vi "save.comics.vi"(8 "error in":errorcluster, 11 "data":T1) -> (0 "error out":errorcluster)   [LabVIEW 2024]
uses:
  TypeDefs/comics.reply--cluster.ctl
  TypeDefs/comic--cluster.ctl
  <vilib>/addons/_JKI.lib/Serialization/JSON/JKI JSON Serialization.lvlib
panel:
  out "all lower case string":string
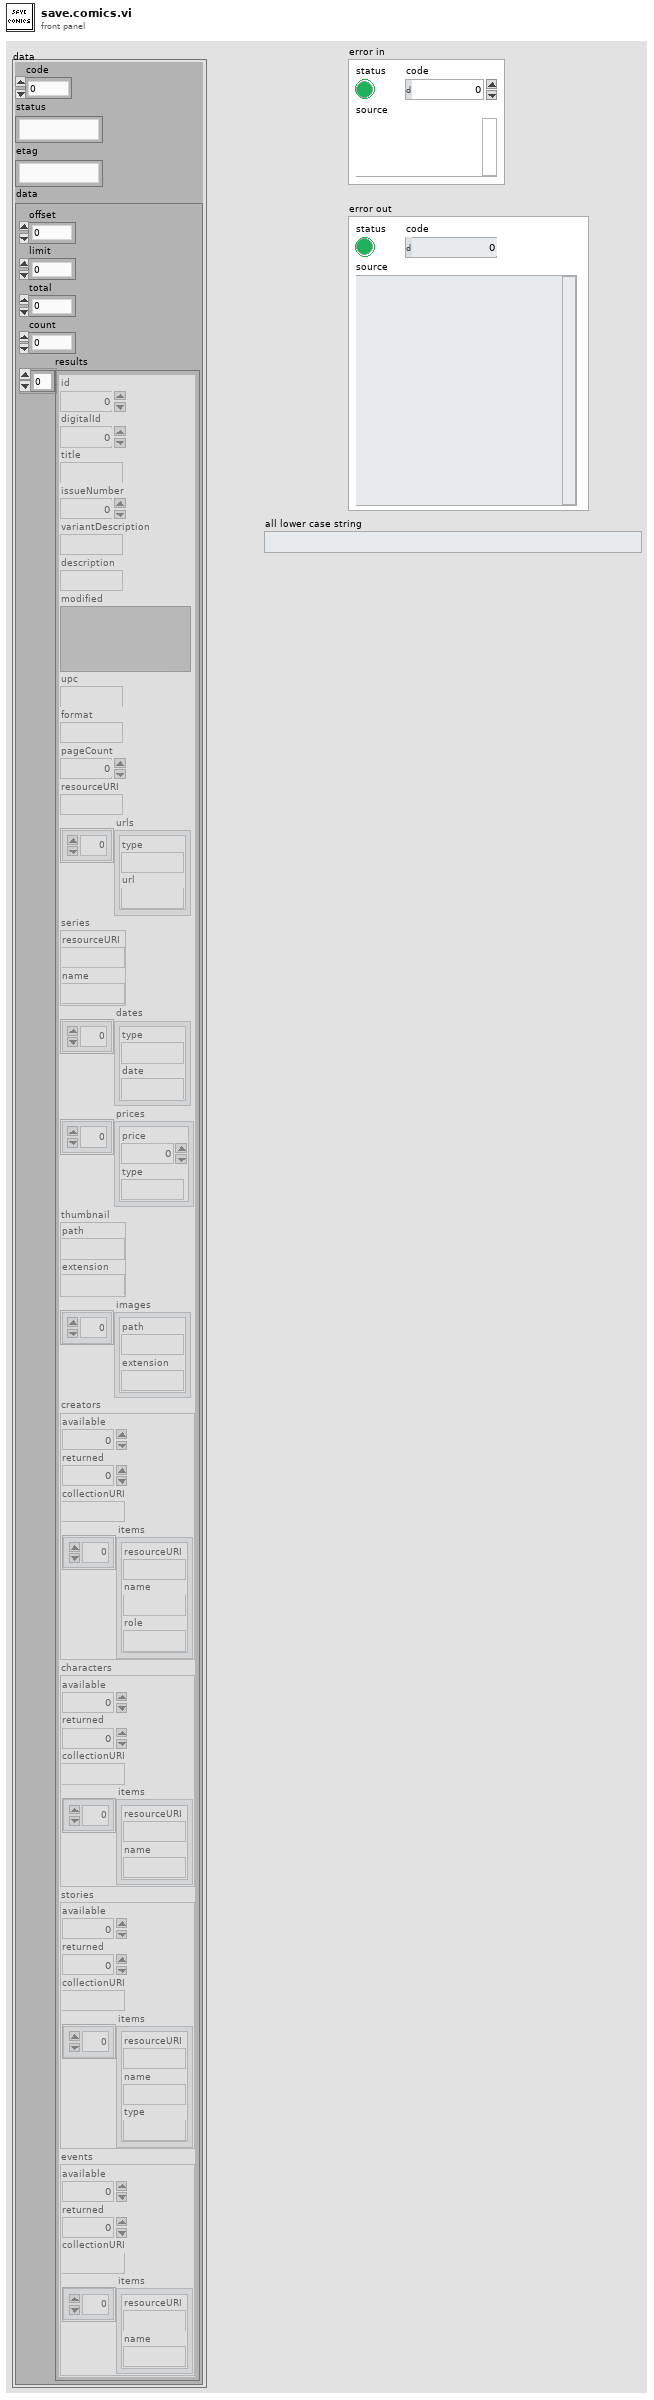
[diagram p1: front panel]
types:
  T1 = typedef "comics.reply--cluster.ctl" = cluster{"code":i32, "status":string, "etag":string, "data":cluster{"offset":i32, "limit":i32, "total":i32, "count":i32, "results":T2[]}}
  T2 = typedef "comic--cluster.ctl" = cluster{"id":i32, "digitalId":i32, "title":string, "issueNumber":i32, "variantDescription":string, "description":string, "modified":variant, "upc":string, "format":string, "pageCount":i32, "resourceURI":string, "urls":cluster{"type":string, "url":string}[], "series":cluster{"resourceURI":string, "name":string}, "dates":cluster{"type":string, "date":string}[], "prices":cluster{"price":dbl, "type":string}[], "thumbnail":cluster{"path":string, "extension":string}, "images":cluster{"path":string, "extension":string}[], "creators":cluster{"available":i32, "returned":i32, "collectionURI":string, "items":cluster{"resourceURI":string, "name":string, "role":string}[]}, "characters":cluster{"available":i32, "returned":i32, "collectionURI":string, "items":cluster{"resourceURI":string, "name":string}[]}, "stories":cluster{"available":i32, "returned":i32, "collectionURI":string, "items":cluster{"resourceURI":string, "name":string, "type":string}[]}, "events":cluster{"available":i32, "returned":i32, "collectionURI":string, "items":cluster{"resourceURI":string, "name":string}[]}}
  T3 = enum16{"open", "replace", "create", "open or create", "replace or create", "replace or create with confirmation"}
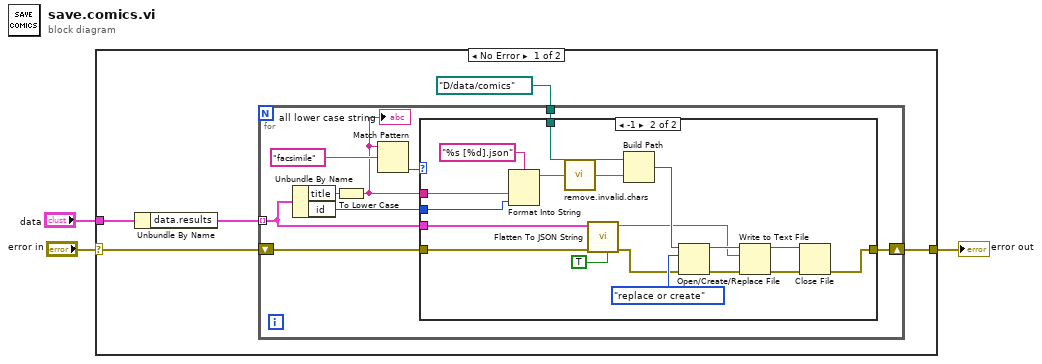
[diagram p0: block diagram]
diagram:
  n1 = case shown="No Error" "error in" {
    selector: "error in" -> [w4 w37]
    tunnel: "data" -> [w8 _]
    tunnel: [w5 w37] -> w2
    frame No Error {
      n2 = Unbundle By Name(w8) -> ("data.results"=w7:T2[])
      n3 = for {
        tunnel: w7 -> [w15] mode=indexing
        tunnel: path "D:/data/comics" ("file (use dialog)") -> [w17]
        shift-right: [w16] -> w5
        shift-left: w4 -> [w14]
        n4 = Unbundle By Name(w15) -> ("title"=w12:string, "id"=w13:i32)
        n5 = To Lower Case(string=w12) -> (all lower case string=w10:string)
        "all lower case string" <- w10
        n6 = Match Pattern(string=w10, regular expression="facsimile") -> (offset past match=w9:i32)  [unwired: 1 in, 3 out]
        n7 = case shown="-1" w9 {
          tunnel: w17 -> [_ w34]
          tunnel: [w18 w27] -> w16
          tunnel: w15 -> [_ w26]
          tunnel: w14 -> [w18 w24]
          tunnel: w13 -> [_ w20]
          tunnel: w10 -> [_ w19]
          frame Default {
          }
          frame -1 {
            n8 = Format Into String(format string="%s [%d].json", w19, w20) -> (resulting string=w35:string)  [unwired: 2 in, 1 out]
            n9 = call "remove.invalid.chars.vi"("string in"=w35) -> ("string out"=w21:string)
            n10 = call <vilib>:"Flatten To JSON String.vi"("Enums As String (F)"=TRUE, "error in (no error)"=w24, "Variant"=w26) -> ("error out"=w23:errorcluster, "JSON String"=w25:string)  [unwired: 7 in]
            n11 = Build Path(base path=w34, name or relative path=w21) -> (appended path=w33:path)
            n12 = Open/Create/Replace File(file path (use dialog)=w33, error in=w23, operation (0:open)=T3."replace or create") -> (refnum out=w31:refnum<file>, error out=w30:errorcluster)  [unwired: 3 in, 1 out]
            n13 = Write to Text File(file (use dialog)=w31, text=w25, error in=w30) -> (refnum out=w28:refnum<file>, error out=w29:errorcluster)  [unwired: 1 in, 1 out]
            n14 = Close File(refnum=w28, error in=w29) -> (error out=w27:errorcluster)  [unwired: 1 out]
          }
        }
      }
    }
    frame Error {
    }
  }
  "error out" <- w2
